vi "Get FIeld Values.vi"(8 "Error in (no error)":errorcluster, 10 "String":string, 11 "Array in":string[](array[string])) -> (0 "Error out":errorcluster, 3 "Array out":dbl[](array[numeric]))   [LabVIEW 2018]
uses:
  <userlib>/caLab/Private/Get_PV-1D.vi
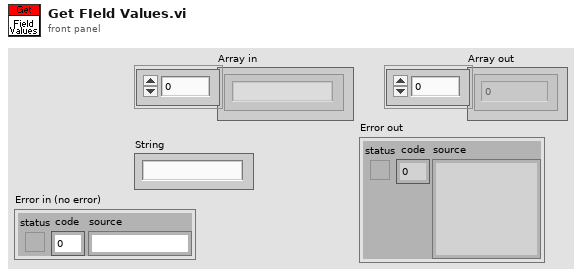
[diagram p1: front panel]
types:
  T1 = typedef "PV Info.ctl" = cluster{"Name":string, "Elements":i32, "Values (string)":string[], "Values (number)":dbl[], "Status (string)":string, "Status (number)":i16, "Severity (string)":string, "Severity (number)":i16, "Timestamp (string)":string, "Timestamp (number)":i32, "Field Names":string[], "Field Values":string[], "Error":errorcluster}
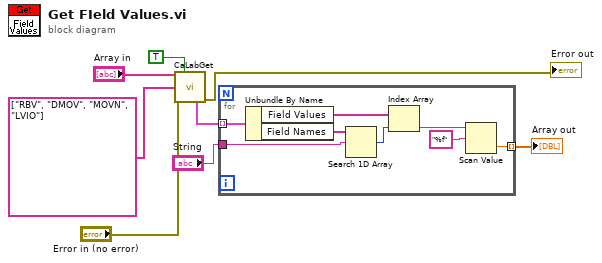
[diagram p0: block diagram]
diagram:
  n1 = call-poly <userlib>:"CaLabGet.vi"("PV Names"="Array in", "variable PV names (F)"=TRUE, "Field Names"=string[] ["RBV", "DMOV", "MOVN", "LVIO"], "Error in (no error)"="Error in (no error)") -> ("PV Info"=w6:T1[], "Error out"=→"Error out":errorcluster)  [unwired: 5 in, 5 out]
  n2 = for {
    tunnel: w6 -> [w16] mode=indexing
    tunnel: "String" -> [w14]
    tunnel: [w10] -> w7 mode=indexing
    n3 = Unbundle By Name(w16) -> ("Field Values"=w12:string[], "Field Names"=w15:string[])
    n4 = Search 1D Array(1D array=w15, element=w14) -> (index of element=w13:i32)  [unwired: 1 in]
    n5 = Index Array(array=w12, index=w13) -> (element=w11:string)
    n6 = Scan Value(string=w11, format string="%f") -> (value=w10:dbl)  [unwired: 1 in, 1 out]
  }
  "Array out" <- w7
